vi "XenaSessions.vi"() -> ()   [LabVIEW 2017]
uses:
  <vilib>/addons/_JKI.lib/REST Client/classes/REST Client/REST Client.lvclass
panel:
  out "Before":string
  out "After":string
  out "resulting string":string
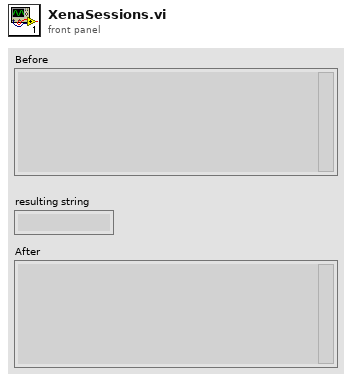
[diagram p1: front panel]
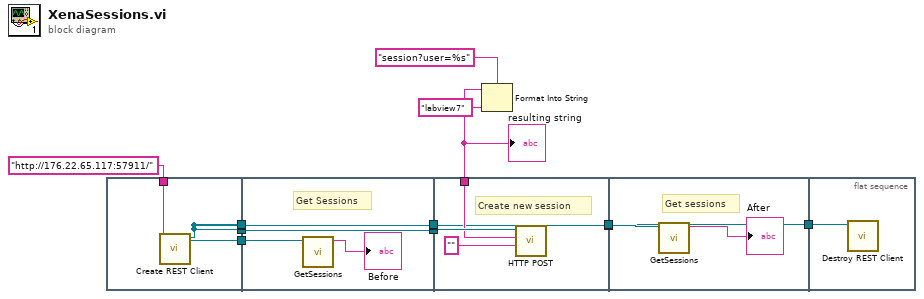
[diagram p0: block diagram]
diagram:
  n1 = flat-sequence {
    tunnel: "http://176.22.65.117:57911/" ("Base URL") -> [w16]
    tunnel: [w15] -> w10
    tunnel: [w15] -> w8
    tunnel: [w15] -> w7
    tunnel: [w15] -> w4
    tunnel: w10 -> [w20]
    tunnel: [w20] -> w9
    tunnel: w8 -> [w19]
    tunnel: w7 -> [w18]
    tunnel: [w18] -> w6
    tunnel: w4 -> [w17]
    tunnel: [w17] -> w3
    tunnel: w11 -> [w25]
    tunnel: w9 -> [w26]
    tunnel: w6 -> [w23]
    tunnel: [w23] -> w5
    tunnel: w3 -> [w22]
    tunnel: [w22] -> w2
    tunnel: w5 -> [w28]
    tunnel: w2 -> [w27]
    tunnel: [w27] -> w1
    tunnel: w1 -> [w30]
    frame #0 {
      n2 = call <vilib>:"Create REST Client.vi"("Base URL"=w16) -> ("REST Client out"=w15:refnum<class "REST Client.lvclass">)  [unwired: 9 in, 1 out]
    }
    frame #1 {
      # "Get Sessions"
      n3 = call "GetSessions.vi"("REST Client in"=w19) -> ("Response body"=→"Before":string)  [unwired: 10 in]
    }
    frame #2 {
      # "Create new session"
      n4 = call-dynamic "HTTP POST.vi"("Request body"="", "Path"=w25, "REST Client in"=w26) -> ()  [unwired: 3 in, 6 out]
    }
    frame #3 {
      # "Get sessions"
      n5 = call "GetSessions.vi"("REST Client in"=w28) -> ("Response body"=→"After":string)  [unwired: 10 in]
    }
    frame #4 {
      n6 = call-dynamic "Destroy REST Client.vi"("REST Client in"=w30) -> ()  [unwired: 10 in, 1 out]
    }
  }
  n7 = Format Into String(format string="session?user=%s", "labview7" ("input 1")) -> (resulting string=w11:string)  [unwired: 2 in, 1 out]
  "resulting string" <- w11
